vi "Test Batch Messaging.vi"(8 "error in":errorcluster, 11 "Test Case In":refnum<class "Messaging Tests.lvclass">) -> (0 "error out":errorcluster, 3 "Test Case Out":refnum<class "Messaging Tests.lvclass">)   [LabVIEW 2020, in "Messaging Tests.lvlib" / "Messaging Tests.lvclass"]
uses:
  Messaging Tests.lvclass
  Messaging Tests.lvclass/Messaging Tests.ctl
  TestActor/Test Actor/TestActor.lvclass
  TestActor/Increment Msg/Increment Msg.lvclass
  vi.lib/ActorFramework/Actor/Actor.lvclass
  vi.lib/ActorFramework/Stop Msg/Stop Msg.lvclass
  vi.lib/ActorFramework/LastAck/Last Ack.lvclass
  vi.lib/ActorFramework/Message Queue/Message Queue.lvclass
  vi.lib/ActorFramework/Message Dequeuer/Message Dequeuer.lvclass
  vi.lib/ActorFramework/Specialty Messages/Batch Msg/Batch Msg.lvclass
  49a6a4ac-6696-4ba8-b226-95e846e01744.vi
  <vilib>/Astemes/LUnit/Test Case.lvclass
  d31e0b00-f115-40d1-b43b-02b0a07bbd24.vi
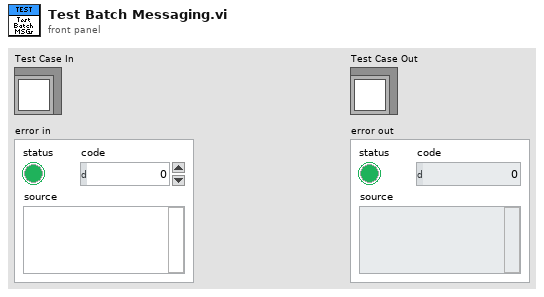
[diagram p1: front panel]
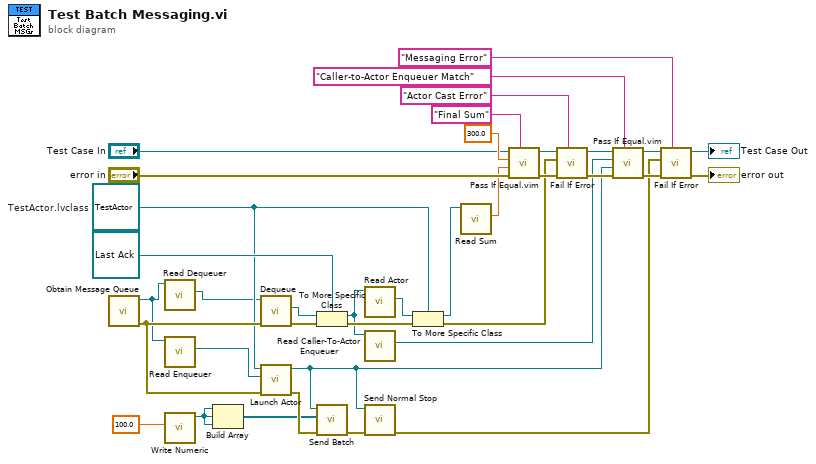
[diagram p0: block diagram]
diagram:
  w23 = refnum<class "TestActor.lvclass"> refnum  # TestActor.lvclass
  n1 = call "Obtain Message Queue.vi"() -> ("error out"=w34:errorcluster, "Message Queue"=w18:refnum<class "Message Queue.lvclass">)  [unwired: 10 in]
  n2 = call "Read Dequeuer.vi"("Message Queue"=w18) -> ("Message Dequeuer"=w16:refnum<class "Message Dequeuer.lvclass">)  [unwired: 10 in]
  n3 = call "Read Enqueuer.vi"("Message Queue"=w18) -> ("Message Enqueuer"=w17:refnum<class "Message Enqueuer.lvclass">)  [unwired: 10 in]
  n4 = call "Write Numeric.vi"("Numeric"=100.0) -> ("Increment Msg out"=w20:refnum<class "Increment Msg.lvclass">)  [unwired: 10 in]
  n5 = Build Array(w20, w20, w20) -> (w19:refnum<class "Increment Msg.lvclass">[])
  n6 = call "Dequeue.vi"("error in (no error)"=w34, "Message Dequeuer in"=w16) -> ("error out"=w33:errorcluster, "Message"=w15:refnum<class "Message.lvclass">)  [unwired: 5 in, 3 out]
  n7 = call "Launch Actor.vi"("error in (no error)"=w34, "Actor-to-Caller Enqueuer"=w17, "Actor"=w23) -> ("error out"=w36:errorcluster, "Caller-To-Actor Enqueuer"=w6:refnum<class "Message Enqueuer.lvclass">)  [unwired: 7 in]
  n8 = To More Specific Class(target class=refnum<class "Last Ack.lvclass"> refnum ("Actor Framework.lvlib:Last Ack"), reference=w15, error in=w33) -> (specific class reference=w14:refnum<class "Last Ack.lvclass">, error out=w37:errorcluster)
  n9 = call "Send Batch.vi"("error in (no error)"=w36, "Messages Array"=w19, "Message Enqueuer"=w6) -> ("error out"=w35:errorcluster)  [unwired: 8 in]
  n10 = call "Read Actor.vi"("Last Ack"=w14) -> ("Actor"=w24:refnum<class "Actor.lvclass">)  [unwired: 10 in]
  n11 = call "Read Caller-To-Actor Enqueuer.vi"("Last Ack"=w14) -> ("Caller-to-Actor Enqueuer"=w7:refnum<class "Message Enqueuer.lvclass">)  [unwired: 10 in]
  n12 = call "Send Normal Stop.vi"("error in (no error)"=w35, "Message Enqueuer"=w6) -> ("error out"=w27:errorcluster)  [unwired: 9 in]
  n13 = To More Specific Class(target class=w23, reference=w24, error in=w37) -> (specific class reference=w22:refnum<class "TestActor.lvclass">, error out=w28:errorcluster)
  n14 = call "Read Sum.vi"("TestActor in"=w22) -> ("Sum"=w10:dbl)  [unwired: 9 in, 1 out]
  n15 = call "Pass If Equal.vim"("Description"="Final Sum", "error in (no error)"="error in", "Actual"=w10, "Expected"=300.0 ("x"), "LUnit Test Case In"="Test Case In") -> ("error out"=w31:errorcluster, "LUnit Test Case Out"=w13:refnum<class "Messaging Tests.lvclass">)  [unwired: 5 in]
  n16 = call <vilib>:"Fail If Error.vi"("Description"="Actor Cast Error", "error in (no error)"=w31, "Assert error"=w28, "LUnit Test Case In"=w13) -> ("error out"=w32:errorcluster, "LUnit Test Case Out"=w12:refnum<class "Messaging Tests.lvclass">)  [unwired: 6 in]
  n17 = call "Pass If Equal.vim"("Description"="Caller-to-Actor Enqueuer Match", "error in (no error)"=w32, "Actual"=w6, "Expected"=w7, "LUnit Test Case In"=w12) -> ("error out"=w30:errorcluster, "LUnit Test Case Out"=w11:refnum<class "Messaging Tests.lvclass">)  [unwired: 5 in]
  n18 = call <vilib>:"Fail If Error.vi"("Description"="Messaging Error", "error in (no error)"=w30, "Assert error"=w27, "LUnit Test Case In"=w11) -> ("error out"=→"error out":errorcluster, "LUnit Test Case Out"=→"Test Case Out":refnum<class "Messaging Tests.lvclass">)  [unwired: 6 in]
